vi "EXECUTION_UI_RESTORE.vi"(8 "error in (no error)":errorcluster, 11 "Main Continer":refnum<vi>) -> (0 "error out":errorcluster)   [LabVIEW 2015, in "Execution.lvclass"]
uses:
  Execution.lvclass
  <vilib>/Utility/miscctls.llb/LVPositionTypeDef.ctl
  <vilib>/Utility/miscctls.llb/LVBoundsTypeDef.ctl
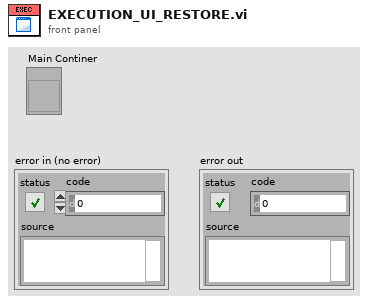
[diagram p1: front panel]
types:
  T1 = typedef "LVPositionTypeDef.ctl" = cluster{"Left":i32, "Top":i32}
  T2 = typedef "LVBoundsTypeDef.ctl" = cluster{"Width":u32, "Height":u32}
  T3 = cluster{"Label.Text":string, "Position":T1, "Container Bounds":T2}[]
  T4 = enum16{"No Scaling", "Scale All Objects", "Scale Single Object"}
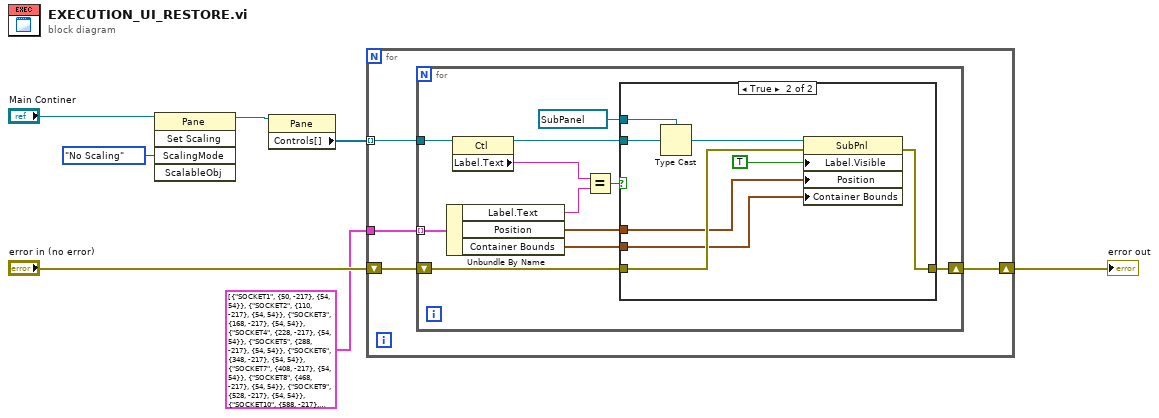
[diagram p0: block diagram]
diagram:
  n1 = invoke class="Pane" method="Set Scaling"(reference="Main Continer", "ScalingMode"=T4."No Scaling" ("Scaling Mode")) -> (reference out=w2:refnum<vi>)  [unwired: 3 in, 4 out]
  n2 = property class="Pane"(reference=w2) -> ("Controls[]"=w5:refnum<vi>[])  [unwired: 1 in, 2 out]
  n3 = for {
    shift-right: [w8] -> w7
    shift-left: "error in (no error)" -> [w11]
    tunnel: w5 -> [w10] mode=indexing
    tunnel: T3 [{"Label.Text"="SOCKET1", "Position"={"Left"=50, "Top"=-217}, "Container Bounds"={"Width"=54, "Height"=54}}, {"Label.Text"="SOCKET2", "Position"={"Left"=110, "Top"=-217}, "Container Bounds"={"Width"=54, "Height"=54}}, {"Label.Text"="SOCKET3", "Position"={"Left"=168, "Top"=-217}, "Container Bounds"={"Width"=54, "Height"=54}}, {"Label.Text"="SOCKET4", "Position"={"Left"=228, "Top"=-217}, "Container Bounds"={"Width"=54, "Height"=54}}, {"Label.Text"="SOCKET5", "Position"={"Left"=288, "Top"=-217}, "Container Bounds"={"Width"=54, "Height"=54}}, {"Label.Text"="SOCKET6", "Position"={"Left"=348, "Top"=-217}, "Container Bounds"={"Width"=54, "Height"=54}}, {"Label.Text"="SOCKET7", "Position"={"Left"=408, "Top"=-217}, "Container Bounds"={"Width"=54, "Height"=54}}, {"Label.Text"="SOCKET8", "Position"={"Left"=468, "Top"=-217}, "Container Bounds"={"Width"=54, "Height"=54}}, {"Label.Text"="SOCKET9", "Position"={"Left"=528, "Top"=-217}, "Container Bounds"={"Width"=54, "Height"=54}}, {"Label.Text"="SOCKET10", "Position"={"Left"=588, "Top"=-217}, "Container Bounds"={"Width"=54, "Height"=54}}, {"Label.Text"="SOCKET11", "Position"={"Left"=648, "Top"=-217}, "Container Bounds"={"Width"=54, "Height"=54}}, {"Label.Text"="SOCKET12", "Position"={"Left"=708, "Top"=-217}, "Container Bounds"={"Width"=54, "Height"=54}}, {"Label.Text"="SOCKET13", "Position"={"Left"=768, "Top"=-217}, "Container Bounds"={"Width"=54, "Height"=54}}, {"Label.Text"="SOCKET14", "Position"={"Left"=828, "Top"=-217}, "Container Bounds"={"Width"=54, "Height"=54}}, {"Label.Text"="SOCKET15", "Position"={"Left"=888, "Top"=-217}, "Container Bounds"={"Width"=54, "Height"=54}}, {"Label.Text"="SOCKET16", "Position"={"Left"=948, "Top"=-217}, "Container Bounds"={"Width"=54, "Height"=54}}, {"Label.Text"="SOCKET17", "Position"={"Left"=50, "Top"=-129}, "Container Bounds"={"Width"=54, "Height"=54}}, {"Label.Text"="SOCKET18", "Position"={"Left"=110, "Top"=-129}, "Container Bounds"={"Width"=54, "Height"=54}}, {"Label.Text"="SOCKET19", "Position"={"Left"=170, "Top"=-129}, "Container Bounds"={"Width"=54, "Height"=54}}, {"Label.Text"="SOCKET20", "Position"={"Left"=230, "Top"=-129}, "Container Bounds"={"Width"=54, "Height"=54}}, {"Label.Text"="SOCKET21", "Position"={"Left"=290, "Top"=-129}, "Container Bounds"={"Width"=54, "Height"=54}}, {"Label.Text"="SOCKET22", "Position"={"Left"=350, "Top"=-129}, "Container Bounds"={"Width"=54, "Height"=54}}, {"Label.Text"="SOCKET23", "Position"={"Left"=410, "Top"=-129}, "Container Bounds"={"Width"=54, "Height"=54}}, {"Label.Text"="SOCKET24", "Position"={"Left"=470, "Top"=-129}, "Container Bounds"={"Width"=54, "Height"=54}}, {"Label.Text"="SOCKET25", "Position"={"Left"=530, "Top"=-129}, "Container Bounds"={"Width"=54, "Height"=54}}, {"Label.Text"="SOCKET26", "Position"={"Left"=590, "Top"=-129}, "Container Bounds"={"Width"=54, "Height"=54}}, {"Label.Text"="SOCKET27", "Position"={"Left"=650, "Top"=-129}, "Container Bounds"={"Width"=54, "Height"=54}}, {"Label.Text"="SOCKET28", "Position"={"Left"=710, "Top"=-129}, "Container Bounds"={"Width"=54, "Height"=54}}, {"Label.Text"="SOCKET29", "Position"={"Left"=770, "Top"=-129}, "Container Bounds"={"Width"=54, "Height"=54}}, {"Label.Text"="SOCKET30", "Position"={"Left"=830, "Top"=-129}, "Container Bounds"={"Width"=54, "Height"=54}}, {"Label.Text"="SOCKET31", "Position"={"Left"=890, "Top"=-129}, "Container Bounds"={"Width"=54, "Height"=54}}, {"Label.Text"="SOCKET32", "Position"={"Left"=950, "Top"=-129}, "Container Bounds"={"Width"=54, "Height"=54}}] ("Array") -> [w9]
    n4 = for {
      shift-right: [w14] -> w8
      shift-left: w11 -> [w15]
      tunnel: w10 -> [w22]
      tunnel: w9 -> [w21] mode=indexing
      n5 = Unbundle By Name(w21) -> ("Label.Text"=w20:string, "Position"=w17:T1, "Container Bounds"=w16:T2)
      n6 = property class="Ctl"(reference=w22) -> (reference out=w18:refnum<vi>, "Label.Text"=w13:string)  [unwired: 1 in, 1 out]
      n7 = Equal?(x=w13, y=w20) -> (x = y?=w19:bool)
      n8 = case shown="True" w19 {
        tunnel: w18 -> [_ w29]
        tunnel: w17 -> [_ w25]
        tunnel: w16 -> [_ w26]
        tunnel: w15 -> [w23 w31]
        tunnel: [w23 w30] -> w14
        tunnel: refnum<vi> refnum ("reference out") -> [_ w27]
        frame False {
        }
        frame True {
          n9 = Type Cast(type=w27, x=w29) -> (*(type *) &x=w28:refnum<vi>)
          n10 = property class="SubPnl"(reference=w28, error in=w31, "Label.Visible"=TRUE, "Position"=w25, "Container Bounds"=w26) -> (error out=w30:errorcluster)  [unwired: 1 out]
        }
      }
    }
  }
  "error out" <- w7
